vi "ACQ 1x summary temp.vi"(3 "1x ChipID list":u16[](array[numeric]) format="%.0x", 4 "ACQtemp* pattern":string, 5 "ACQ full DATA file path":path caption="File path") -> (1 "1x summary temp out":u32[][](array[numeric]))   [LabVIEW 2015, in "VIPM2.lvlib"]
doc: "Genera summary d'una FPGA amb tots els seus ACQtemp*."
uses:
  VIPM2.lvlib
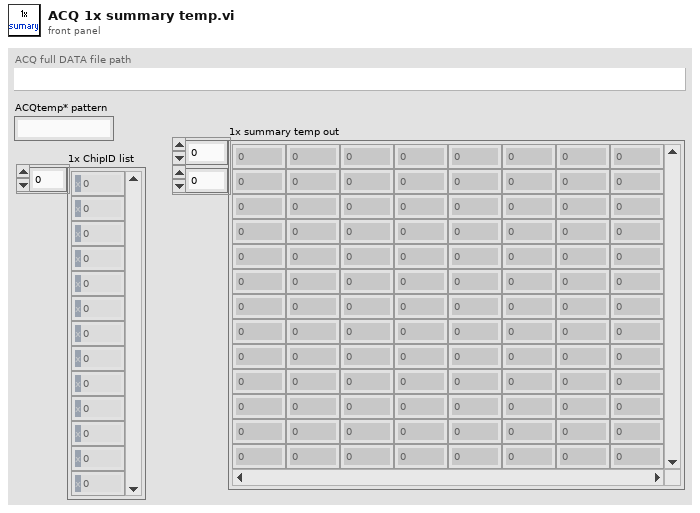
[diagram p1: front panel]
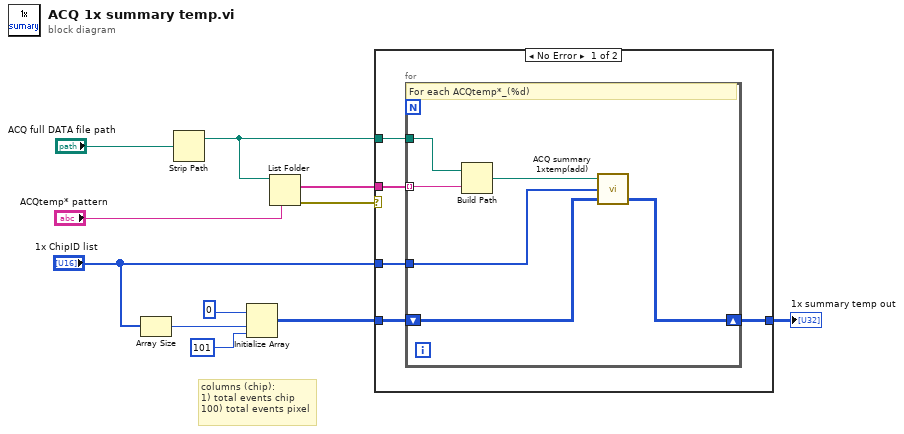
[diagram p0: block diagram]
diagram:
  # "columns (chip):\n1) total events chip\n100) total events pixel"
  n1 = Array Size(array="1x ChipID list") -> (size(s)=w4:i32)
  n2 = Strip Path(path="ACQ full DATA file path") -> (stripped path=w7:path)  [unwired: 1 out]
  n3 = Initialize Array "Initialize Array"(u32 0 ("element"), w4, 101 ("dimension size")) -> (w2:u32[][])
  n4 = List Folder(path=w7, pattern="ACQtemp* pattern") -> (filenames=w8:string[], error out=w9:errorcluster)  [unwired: 2 in, 2 out]
  n5 = case shown="No Error" w9 {
    tunnel: w8 -> [w16 _]
    tunnel: w7 -> [w15 _]
    tunnel: "1x ChipID list" -> [w14 _]
    tunnel: w2 -> [w13 w23]
    tunnel: [w12 w23] -> w1
    frame No Error {
      n6 = for {
        tunnel: w16 -> [w22] mode=indexing
        tunnel: w15 -> [w21]
        tunnel: w14 -> [w19]
        shift-right: [w17] -> w12
        shift-left: w13 -> [w18]
        # "For each ACQtemp*_(%d)"
        n7 = Build Path(base path=w21, name or relative path=w22) -> (appended path=w20:path)
        n8 = call "ACQ summary 1xtemp(add).vi"("temp summary in"=w18, "ChipID list"=w19, "ACQtemp file path in"=w20) -> ("temp summary out"=w17:u32[][])  [unwired: 2 in]
      }
    }
    frame Error {
    }
  }
  "1x summary temp out" <- w1
